vi "beräknaS.vi"(11 "medelvärde":dbl[][](array[numeric])) -> (1 "E-värden":dbl[](array[numeric]), 2 "S-värde":dbl format="%.2f")   [LabVIEW 2020]
uses:
  <vilib>/Analysis/baseanly.llb/Real Dot Product.vi
  <vilib>/Analysis/NI_AALBase.lvlib
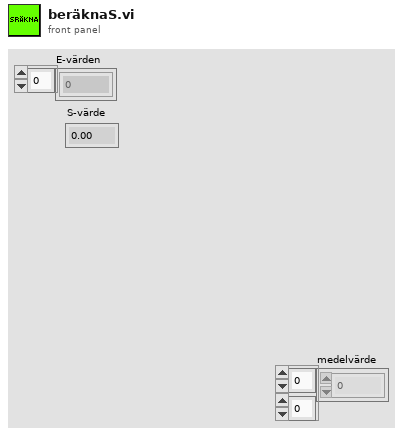
[diagram p1: front panel]
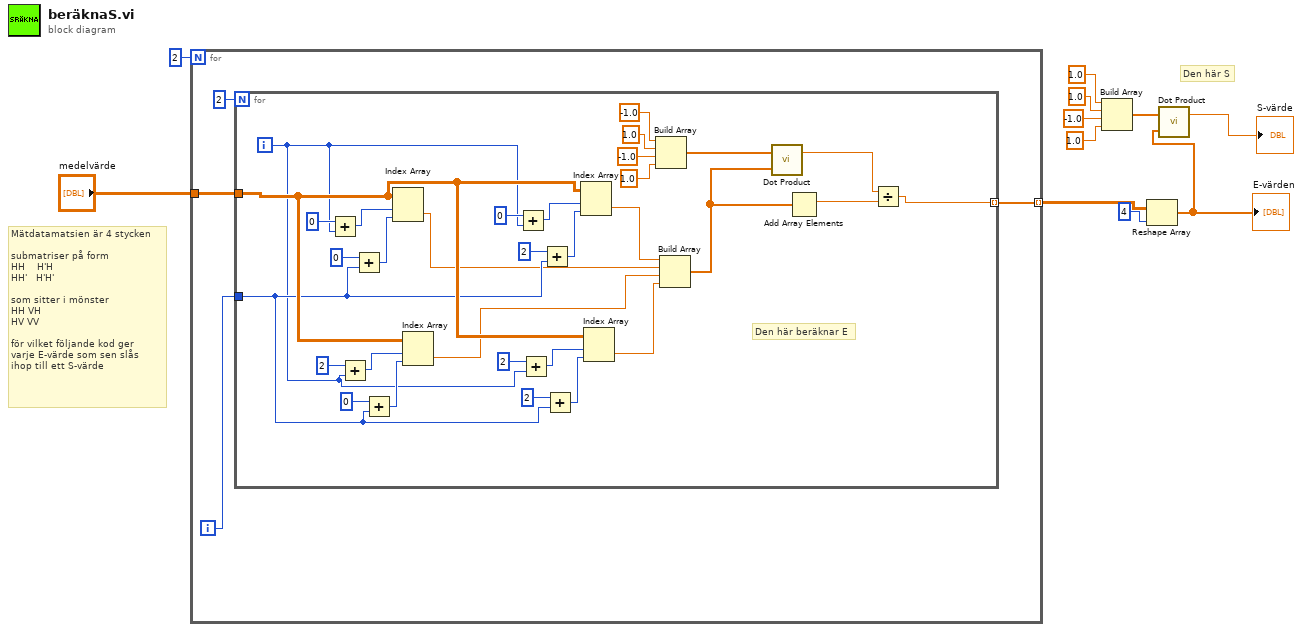
[diagram p0: block diagram]
diagram:
  # "Den här S"
  # "Mätdatamatsien är 4 stycken \n\nsubmatriser på form \nHH    H'H\nHH'   H'H'\n\nsom sitter i mönster \nHH VH\nHV VV\n\nför vilket följande kod ger \nvarje E-värde som sen slås \nihop till ett S-värde"
  n1 = for {
    N: 2 -> [_]
    tunnel: "medelvärde" -> [w15]
    tunnel: [w13] -> w5 mode=indexing
    i -> [w14]
    n2 = for {
      N: 2 -> [_]
      tunnel: w15 -> [w31]
      tunnel: w14 -> [w30]
      tunnel: [w18] -> w13 mode=indexing
      i -> [w29]
      # "Den här beräknar E"
      n3 = Add(x=0 ("index (row)"), y=w29) -> (x+y=w47:i32)
      n4 = Add(x=2 ("index (row)"), y=w29) -> (x+y=w43:i32)
      n5 = Add(x=0 ("index (row)"), y=w30) -> (x+y=w44:i32)
      n6 = Add(x=0 ("index (row)"), y=w30) -> (x+y=w40:i32)
      n7 = Index Array(array=w31, index (row)=w47, index (col)=w44) -> (element=w27:dbl)
      n8 = Index Array(array=w31, index (row)=w43, index (col)=w40) -> (element=w26:dbl)
      n9 = Add(x=0 ("index (row)"), y=w29) -> (x+y=w39:i32)
      n10 = Add(x=2 ("index (row)"), y=w29) -> (x+y=w35:i32)
      n11 = Add(x=2 ("index (row)"), y=w30) -> (x+y=w36:i32)
      n12 = Add(x=2 ("index (row)"), y=w30) -> (x+y=w32:i32)
      n13 = Index Array(array=w31, index (row)=w39, index (col)=w36) -> (element=w28:dbl)
      n14 = Index Array(array=w31, index (row)=w35, index (col)=w32) -> (element=w25:dbl)
      n15 = Build Array(-1.0 ("element"), 1.0 ("element"), -1.0 ("element"), 1.0 ("element")) -> (w16:dbl[])
      n16 = Build Array(w28, w27, w26, w25) -> (w17:dbl[])
      n17 = call-poly <vilib>:"Dot Product.vi"("Y Vector"=w17, "X Vector"=w16) -> ("X * Y"=w19:dbl)  [unwired: 1 out]
      n18 = Add Array Elements(numeric array=w17) -> (sum=w20:dbl)
      n19 = Divide(x=w19, y=w20) -> (x/y=w18:dbl)
    }
  }
  n20 = Build Array(1.0 ("element"), 1.0 ("element"), -1.0 ("element"), 1.0 ("element")) -> (w4:dbl[])
  n21 = Reshape Array(w5, 4 ("dimension size")) -> (w2:dbl[])
  "E-värden" <- w2
  n22 = call-poly <vilib>:"Dot Product.vi"("Y Vector"=w2, "X Vector"=w4) -> ("X * Y"=→"S-värde":dbl)  [unwired: 1 out]
